vi "Port Close (SubVI).vi"(2 "error in":errorcluster, 3 "VISA Refnum in":refnum<visa-resource-name>) -> (0 "error out":errorcluster, 1 "VISA Refnum out":refnum<visa-resource-name>)   [LabVIEW 2017]
doc: "Close the port from a VISA Refnum.\nFlush the buffers and close the VISA session.\nDisplay an error if there is one.\nMade by Tanguy BOULARD\nTHALES FRANCE"
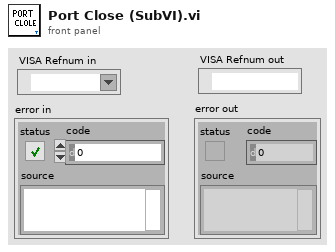
[diagram p1: front panel]
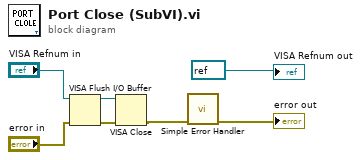
[diagram p0: block diagram]
diagram:
  n1 = VISA Flush I/O Buffer(VISA resource name="VISA Refnum in", error in (no error)="error in") -> (VISA resource name out=w3:refnum<visa-resource-name>, error out=w4:errorcluster)  [unwired: 1 in]
  n2 = VISA Close(VISA resource name=w3, error in (no error)=w4) -> (error out=w6:errorcluster)
  n3 = call <vilib>:"Simple Error Handler.vi"("error in (no error)"=w6) -> ("error out"=→"error out":errorcluster)  [unwired: 4 in, 4 out]
  "VISA Refnum out" <- refnum<visa-resource-name> refnum ("VISA resource Out")
